vi "Read Legend Visible.vi"(8 "error in (no error)":errorcluster, 11 "WaveformGraph.lvclass in":refnum<class "WaveformGraph.lvclass">) -> (0 "error out":errorcluster, 2 "LegVis":bool, 3 "WaveformGraph.lvclass out":refnum<class "WaveformGraph.lvclass">)   [LabVIEW 2015, in "WaveformGraph.lvclass"]
doc: "Shows the plot legend.\n\nQControl Class wrapper around the <b>WaveformGraph : Legend : Visible Property</b>.\n<b> </b> <b> </b>\n©2016 Q Software Innovations, LLC (QSI)\nwritten by Quentin Alldredge\nproduced in LabVIEW 2015\n\nsupport@qsoftwareinnovations.com\nwww.qsoftwareinnovations.com\n\nAll rights reserved.\n\nRedistribution and use in source and binary forms, with or without modification, are permitted provided that the following conditions are met:\n\n * Redistributions of source code must retain the above copyright notice, this list of conditions and the following disclaimer.\n * Redistributions in binary form must reproduce the above copyright notice, this list of conditions and the following disclaimer in the documentation and/or other materials provided with the distribution.\n * Neither the name of Q Software Innovations, LLC. nor the names of its contributors may be used to endorse or promote products derived from this software without specific prior written permission.\n\nTHIS SOFTWARE IS PROVIDED BY THE COPYRIGHT HOLDERS AND CONTRIBUTORS \"AS IS\" AND ANY EXPRESS OR IMPLIED WARRANTIES, INCLUDING, BUT NOT LIMITED TO, THE IMPLIED WARRANTIES OF MERCHANTABILITY AND FITNESS FOR A PARTICULAR PURPOSE ARE DISCLAIMED. IN NO EVENT SHALL THE COPYRIGHT OWNER OR CONTRIBUTORS BE LIABLE FOR ANY DIRECT, INDIRECT, INCIDENTAL, SPECIAL, EXEMPLARY, OR CONSEQUENTIAL DAMAGES (INCLUDING, BUT NOT LIMITED TO, PROCUREMENT OF SUBSTITUTE GOODS OR SERVICES; LOSS OF USE, DATA, OR PROFITS; OR BUSINESS INTERRUPTION) HOWEVER CAUSED AND ON ANY THEORY OF LIABILITY, WHETHER IN CONTRACT, STRICT LIABILITY, OR TORT (INCLUDING NEGLIGENCE OR OTHERWISE) ARISING IN ANY WAY OUT OF THE USE OF THIS SOFTWARE, EVEN IF ADVISED OF THE POSSIBILITY OF SUCH DAMAGE."
uses:
  WaveformGraph.lvclass
  WaveformGraph.lvclass/WaveformGraph.ctl
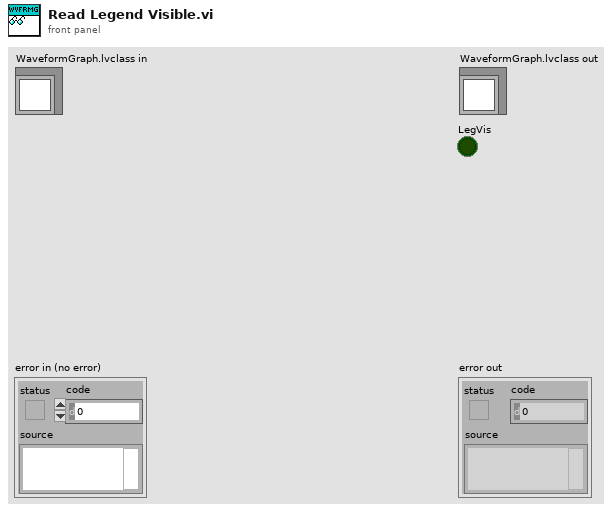
[diagram p1: front panel]
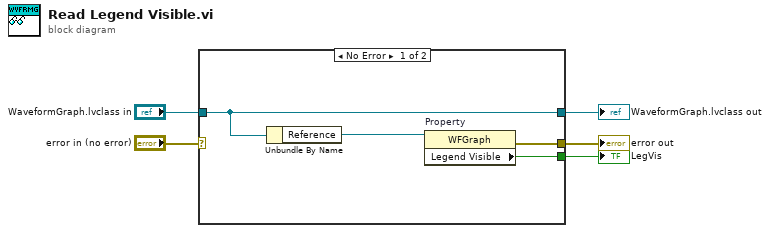
[diagram p0: block diagram]
diagram:
  n1 = case shown="No Error" "error in (no error)" {
    selector: "error in (no error)" -> [_ w11]
    tunnel: [w8 w11] -> w4
    tunnel: [w7 w10] -> w2
    tunnel: "WaveformGraph.lvclass in" -> [w7 w10]
    tunnel: [w9 _] -> w1
    frame No Error {
      n2 = Unbundle By Name(w7) -> ("Reference"=w6:refnum<vi>)
      n3 = property on="Property" class="WFGraph"(reference=w6) -> (error out=w8:errorcluster, "Legend Visible"=w9:bool)  [unwired: 1 in, 1 out]
    }
    frame Error {
    }
  }
  "error out" <- w4
  "WaveformGraph.lvclass out" <- w2
  "LegVis" <- w1
